vi "SubVI_Overlay Circle.vi"(6 "圓標示顏色":u32(colorbox)=3381759, 7 "Group":string, 9 "直徑":dbl=27.742323698834134, 10 "圓心":cluster{"X":sgl, "Y":sgl}, 11 "Image":T1) -> (3 "Image Out":T1)   [LabVIEW 2013]
uses:
  <vilib>/vision/Image Controls.llb/IMAQ Image.ctl
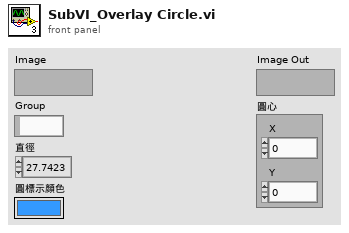
[diagram p1: front panel]
types:
  T1 = typedef "IMAQ Image.ctl" = refnum<image>
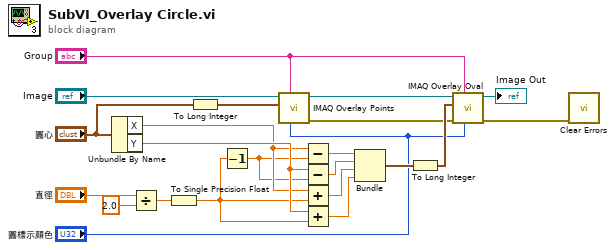
[diagram p0: block diagram]
diagram:
  n1 = Unbundle By Name("圓心") -> ("X"=w15:sgl, "Y"=w16:sgl)
  n2 = Divide(x="直徑", y=2.0) -> (x/y=w3:dbl)
  n3 = To Single Precision Float(number=w3) -> (single precision float=w7:sgl)
  n4 = To Long Integer(number="圓心") -> (32bit integer=w14:cluster{"X":i32, "Y":i32})
  n5 = Decrement(x=w7) -> (x-1=w12:sgl)
  n6 = call "IMAQ Overlay Points"("Color"="圓標示顏色", "Group"="Group", "Point"=w14, "Image"="Image") -> ("error out"=w2:errorcluster, "Image Out"=w13:T1)  [unwired: 6 in]
  n7 = Subtract(x=w15, y=w12) -> (x-y=w17:sgl)
  n8 = Subtract(x=w16, y=w12) -> (x-y=w18:sgl)
  n9 = Add(x=w15, y=w7) -> (x+y=w19:sgl)
  n10 = Add(x=w16, y=w7) -> (x+y=w20:sgl)
  n11 = Bundle(w17, w18, w19, w20) -> (w21:cluster{sgl, sgl, sgl, sgl})  [unwired: 1 in]
  n12 = To Long Integer(number=w21) -> (32bit integer=w22:cluster{i32, i32, i32, i32})
  n13 = call "IMAQ Overlay Oval"("Color"="圓標示顏色", "Group"="Group", "error in (no error)"=w2, "Bounding Rectangle"=w22, "Image"=w13) -> ("error out"=w1:errorcluster, "Image Out"=→"Image Out":T1)  [unwired: 5 in]
  n14 = call <vilib>:"Clear Errors.vi"("error in (no error)"=w1) -> ()  [unwired: 6 in, 1 out]
